vi "DimostratoreCalibrazioni.vi"() -> ()   [LabVIEW 2019]
uses:
  TypeDef/SlugExpiration.ctl
  ByteGSAPIBase/ByteGSAPIBase.lvclass
  TypeDef/CalibrationStates.ctl
  ByteGSAPIBase/FetchCalibration/Converted_Slug_Cluster.ctl
  ByteGSAPIBase/Instruments/Instruments.ctl
  ByteGSAPIBase/CalibrationMeasurements/BodyCalibrazioneMisure.ctl
  aa47c742-c095-4670-bf1f-6b28e4309cef.vi
  <vilib>/numeric/Random Number (Range) I64.vi
  <vilib>/Array/Sort 2D Array - Pop Stack.vi
  <vilib>/Array/Sort 2D Array - Push Stack.vi
  <vilib>/numeric/sub_Random U32.vi
panel:
  in  "Exit":bool
  out "Calibrations":string
  out "Stato":string
  out "Misurazione n.":string
  in  "Cancel":bool
  in  "Approvation":bool
  in  "Avanti":bool
  in  "Repeat":bool
  out "Esito":string
  out "Valore misurato":dbl
  out "Valore di riferimento":dbl
  out "Waveform Chart":i64(graph)
  in  "Start Calibration":bool
  in  "Next":bool
  in  "Previus":bool
  out "Taratura n.":string
  in  "Filtro":enum16{"All", "Expired", "Not Expired"}(ring)
  in  "Slug list":T1[](array[typedef])
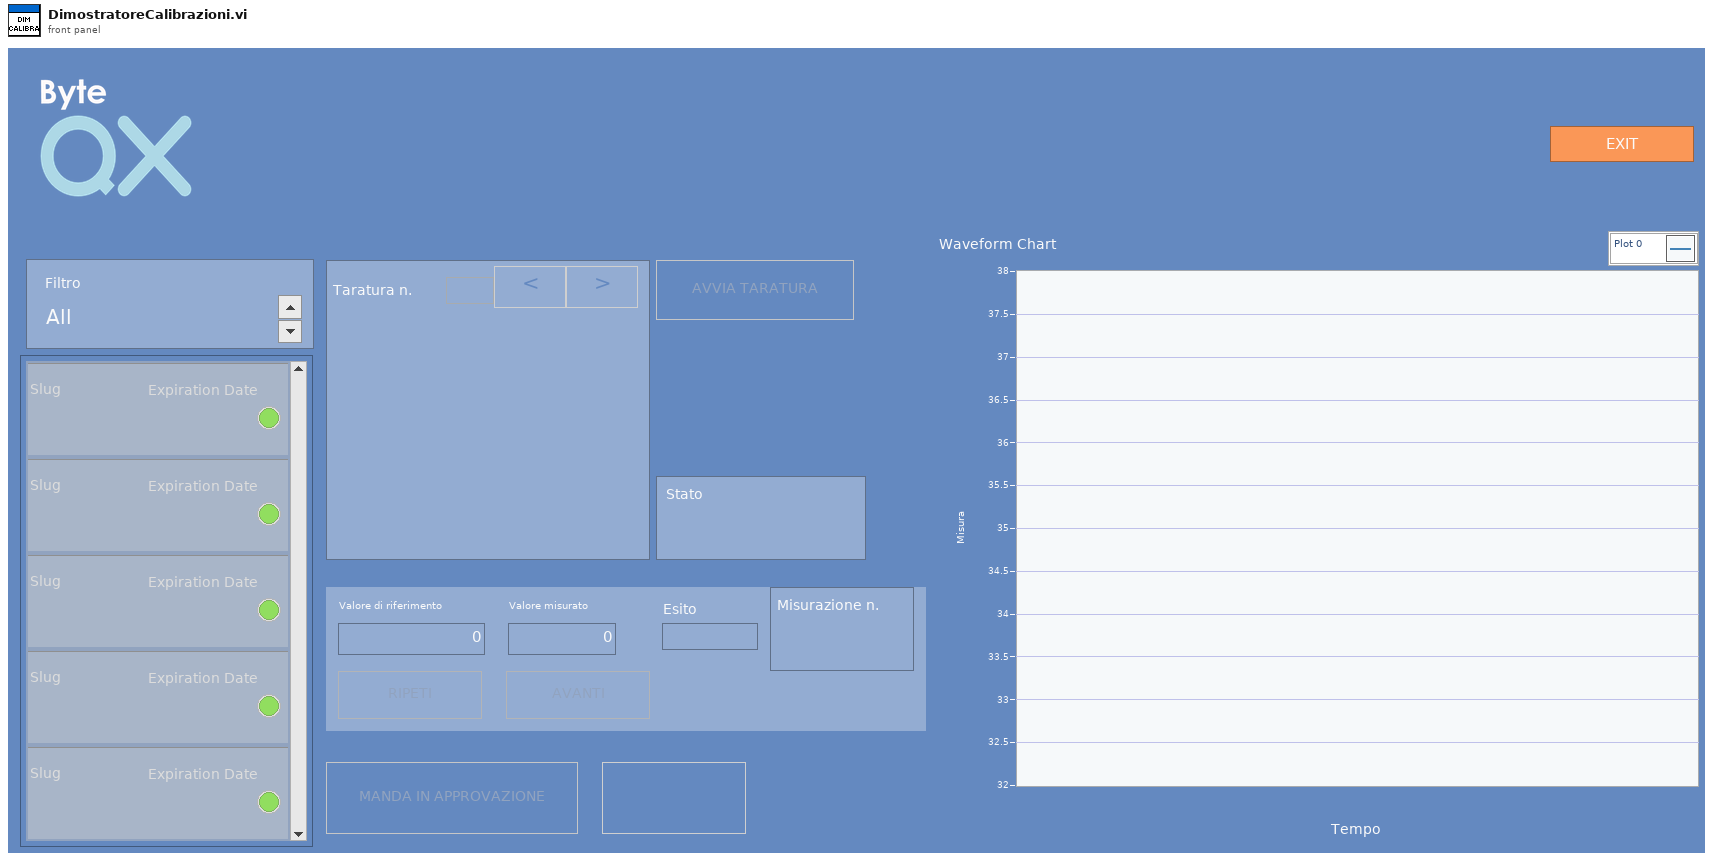
[diagram p1: front panel]
types:
  T1 = typedef "SlugExpiration.ctl" = cluster{"Slug":string, "Expiration Date":string, "Color Box":u32, "Active":bool, "Expired?":bool, "Id":i32}
  T2 = typedef "CalibrationStates.ctl" = enum16{"Init", "Idle", "GetInstruments", "Fetch", "GetCalibrations", "CheckTotalMisurations", "StartCalibration", "ManageCalibration", "AllowApprove", "Approve"}
  T3 = typedef "ByteGSWebAPI.lvlib/ByteGSAPIBase.lvclass/BodyCalibrazioneMisure.ctl" = cluster{"controls":cluster{"id":u16, "descrizione":string, "numero_misure_necessarie":u16, "riferimento_obiettivo":dbl, "mpe_max":dbl, "mpe_min":dbl, "deviazione_standard":dbl, "incertezza":dbl, "numero_misure_effettuate":u32, "temperatura_c":dbl, "umidita":dbl, "strumento_riferimento":cluster{"id":u16, "nome":string}[]}[]}
  T4 = typedef "Instruments.ctl" = cluster{"id":i32, "slug":string, "stabilimento":cluster{"id":dbl}, "categoria":cluster{"id":dbl}, "tipologia_di_visualizzazione":cluster{"id":dbl}, "stato":cluster{"id":dbl}, "descrizione":string, "costruttore":string, "matricola":string, "data_registrazione":string, "intervallo_di_taratura_mesi":dbl, "reparto":string, "campo_misura":string, "risoluzione":dbl, "responsabile_strumento":string, "classe_di_precisione":string, "classificazione":string, "appunti":string, "manuale":string, "foto":string, "riferimento":bool, "qr_hashcode":string, "costo_euro":dbl}
  T5 = typedef "ByteGSWebAPI.lvlib/ByteGSAPIBase.lvclass/Converted_Slug_Cluster.ctl" = cluster{"id":u32, "instrument":string, "name":string, "date":timestamp}
  T6 = cluster{"Esito":refnum<vi>, "Avanti":refnum<vi>, "Repeat":refnum<vi>, "Slug list":refnum<vi>, "Start Calibration":refnum<vi>, "Avanti":refnum<vi>, "Cancel":refnum<vi>, "Approvation":refnum<vi>}
  T7 = cluster{"ByteGSAPIBase in":refnum<class "ByteGSAPIBase.lvclass">, "Instruments_Slug":string[], "All_Instruments_Cals":T5[], "All_Instruments":T4[], "Slug list All":T1[], "Calibrations":T3, "Selected Slug":i32, "Misurazioni":string, "Misurazioni index":i32, "Next State":T2, "Waveform Chart":refnum<vi>, "New Val":dbl, "Id Failed":u32, "Failed?":bool, "Cal Index":i32, "Misurazioni n":string, "Stato":string, "Esito":string, "Misure effettuate":i32, "Calibrations":string}
  T8 = cluster{"id":u16, "descrizione":string, "numero_misure_necessarie":u16, "riferimento_obiettivo":dbl, "mpe_max":dbl, "mpe_min":dbl, "deviazione_standard":dbl, "incertezza":dbl, "numero_misure_effettuate":u32, "temperatura_c":dbl, "umidita":dbl, "strumento_riferimento":cluster{"id":u16, "nome":string}[]}[]
  T9 = cluster{"id":u16, "descrizione":string, "numero_misure_necessarie":u16, "riferimento_obiettivo":dbl, "mpe_max":dbl, "mpe_min":dbl, "deviazione_standard":dbl, "incertezza":dbl, "numero_misure_effettuate":u32, "temperatura_c":dbl, "umidita":dbl, "strumento_riferimento":cluster{"id":u16, "nome":string}[]}
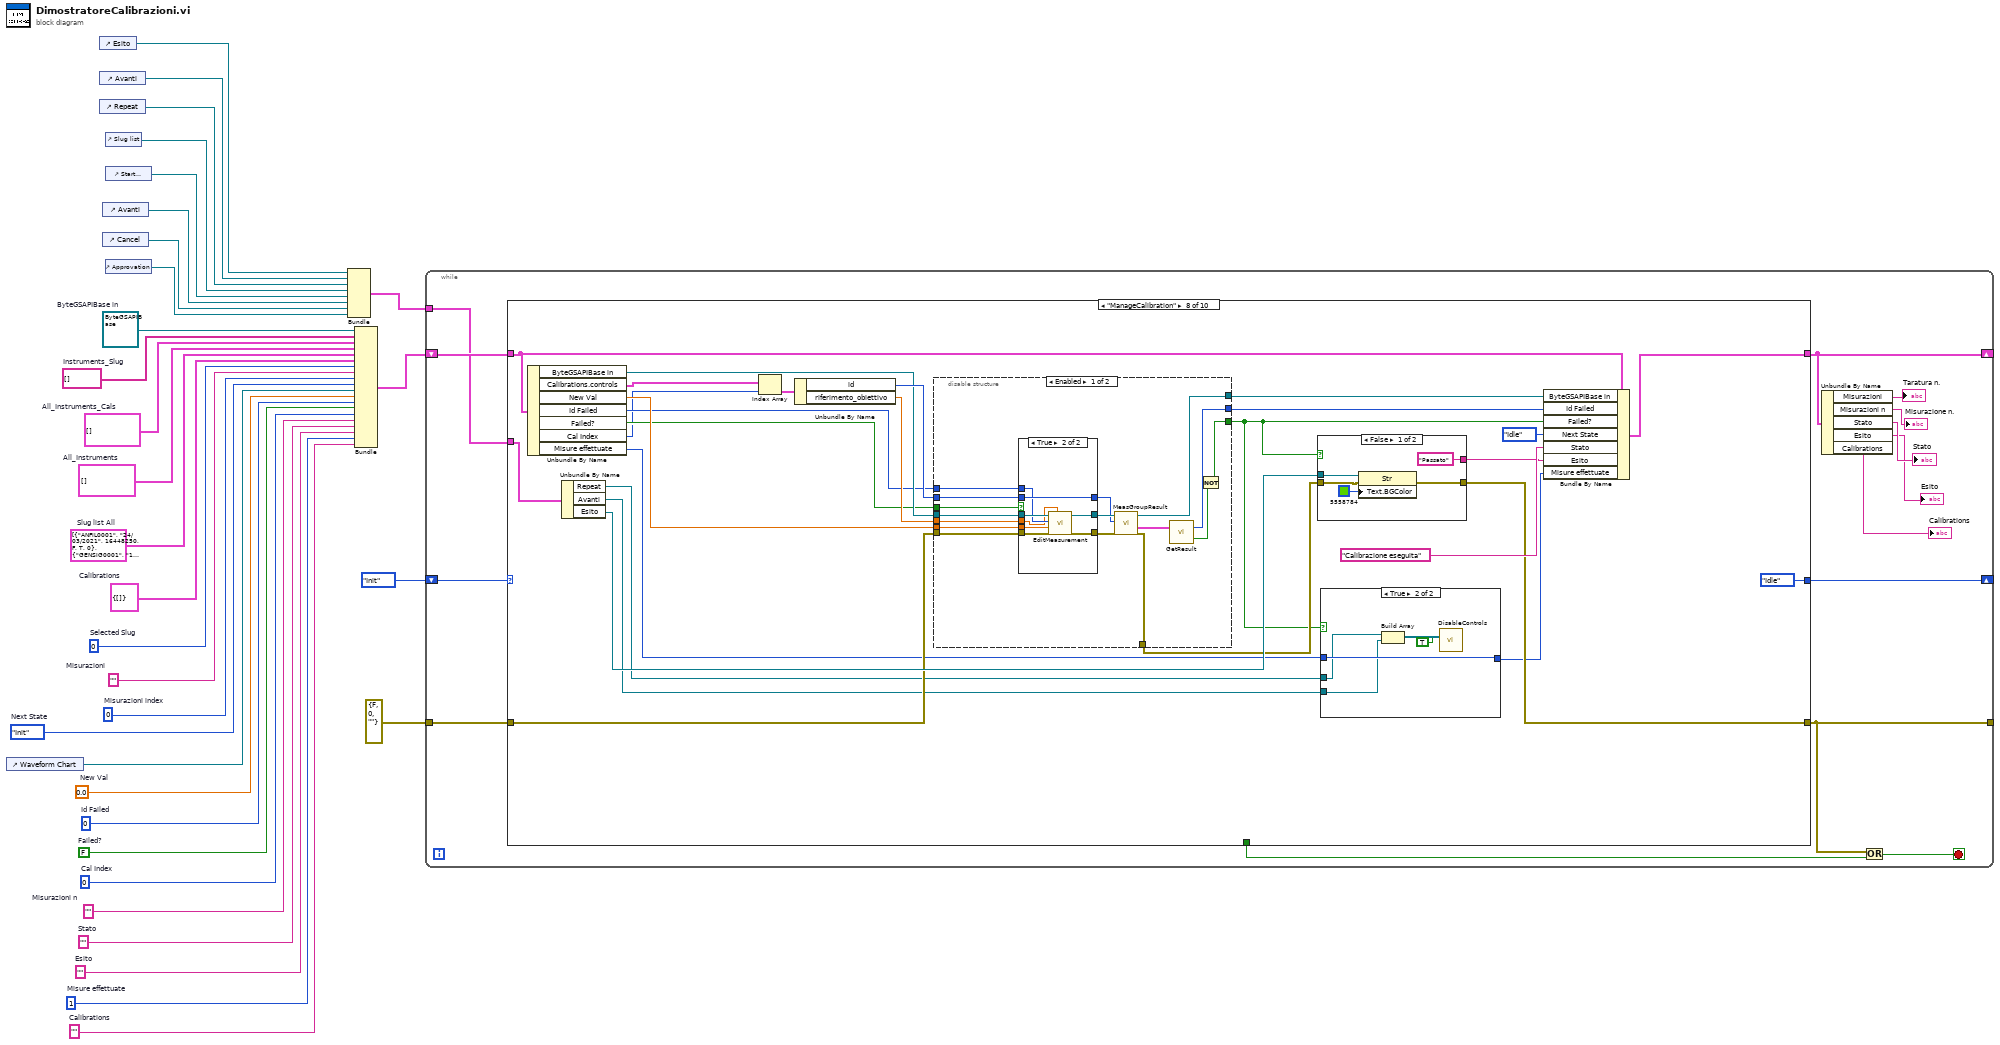
[diagram p0: block diagram]
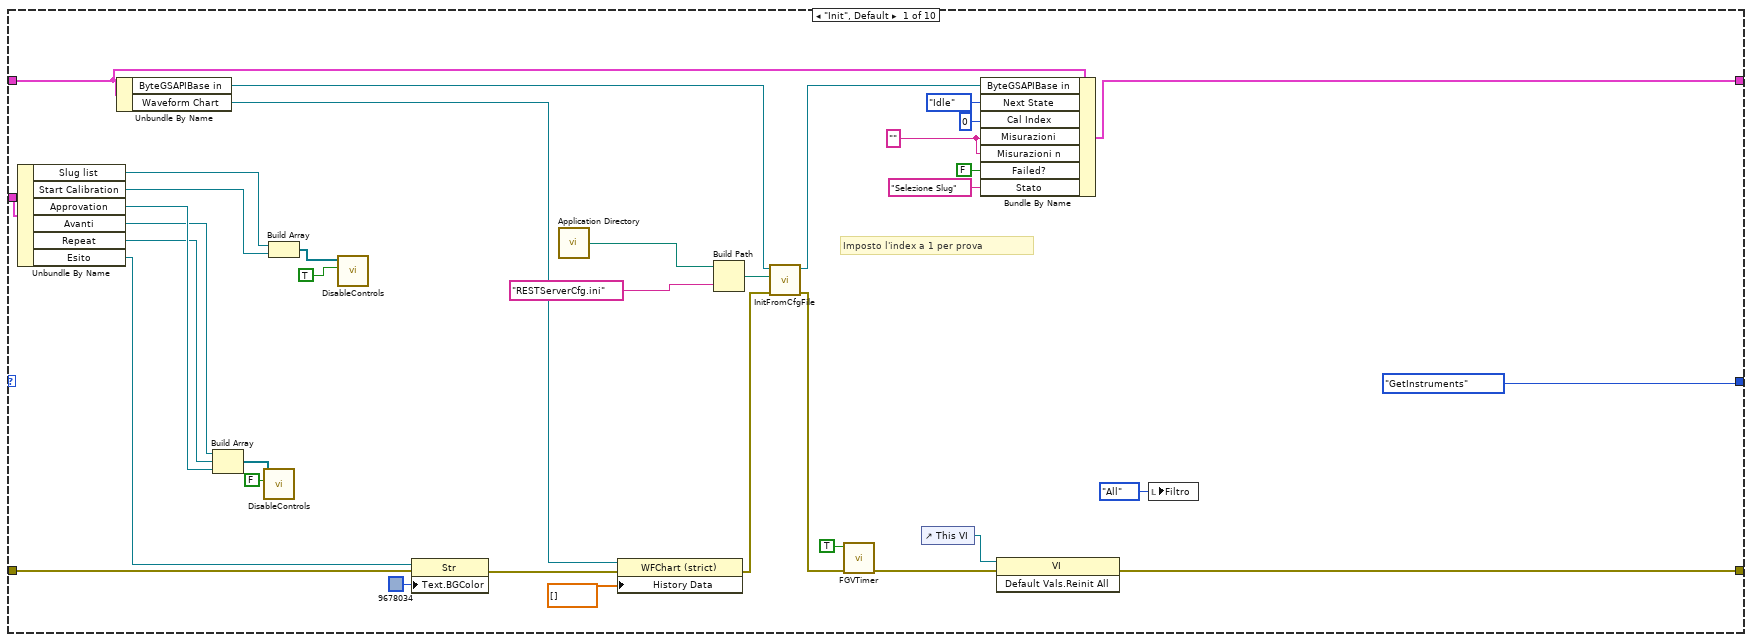
[diagram p2: hidden frame]
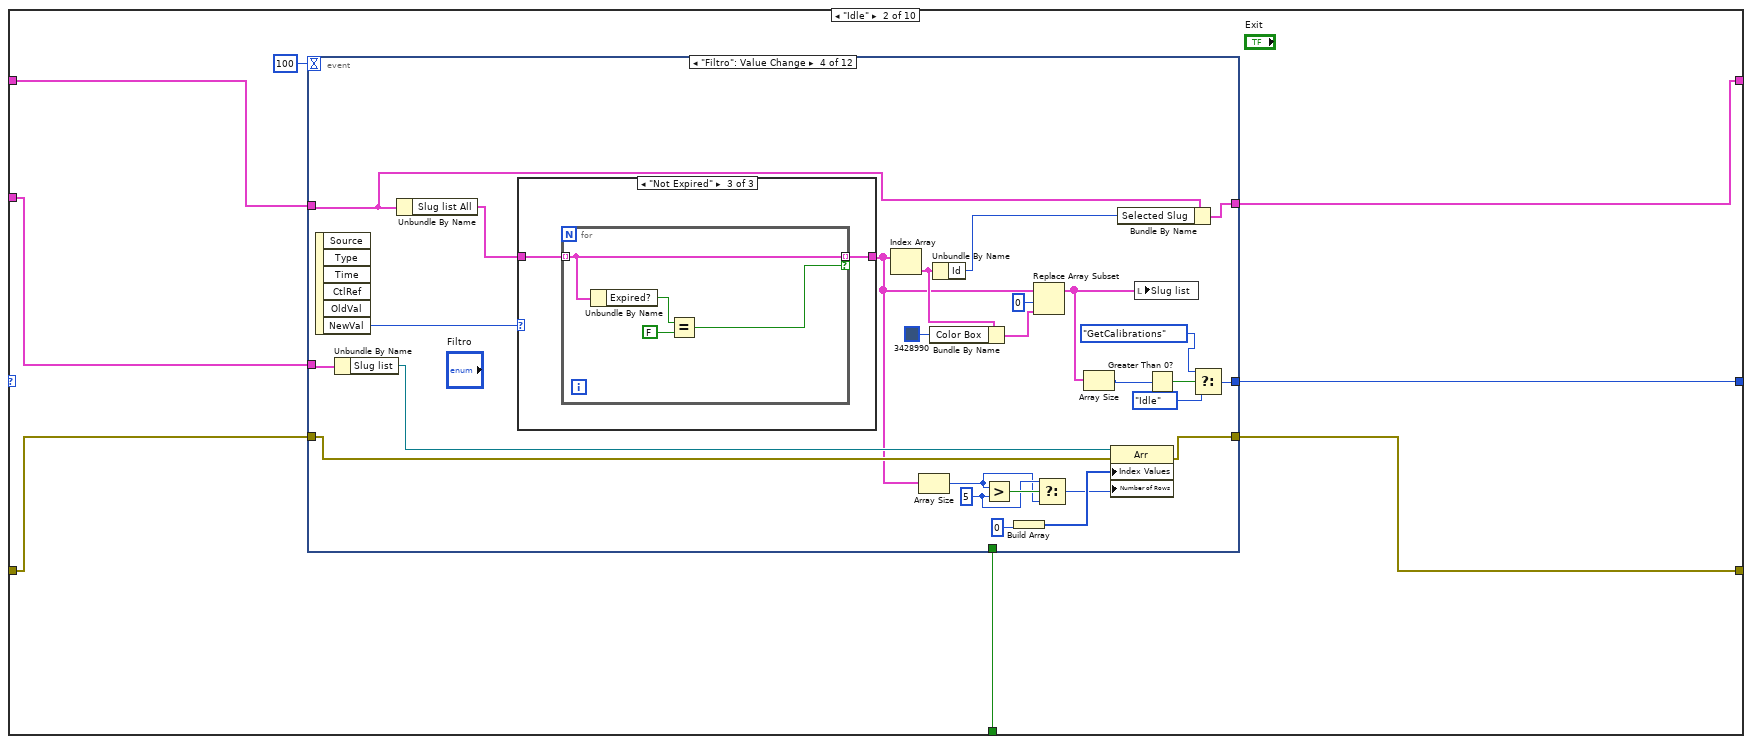
[diagram p3: hidden frame]
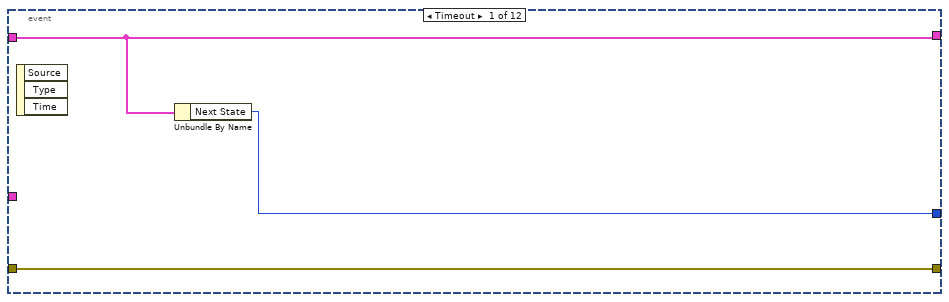
[diagram p4: hidden frame]
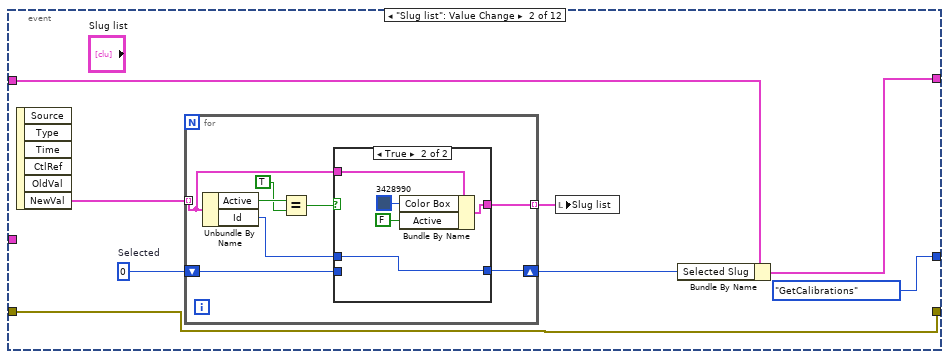
[diagram p5: hidden frame]
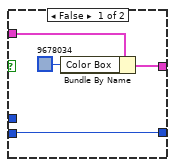
[diagram p6: hidden frame]
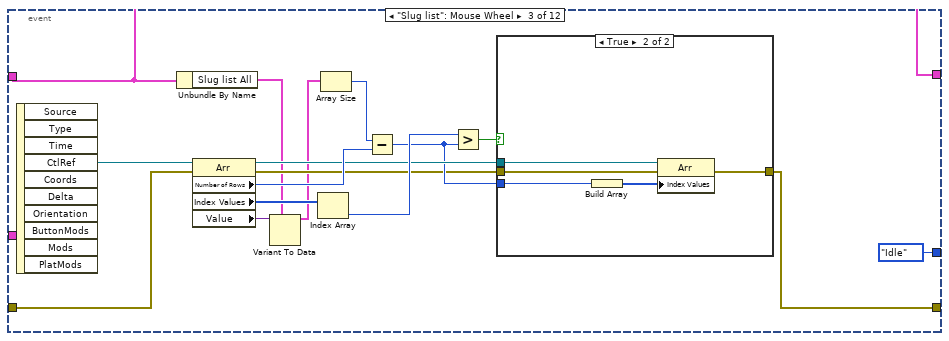
[diagram p7: hidden frame]
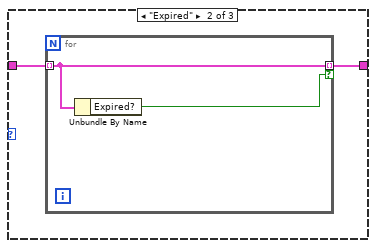
[diagram p10: hidden frame]
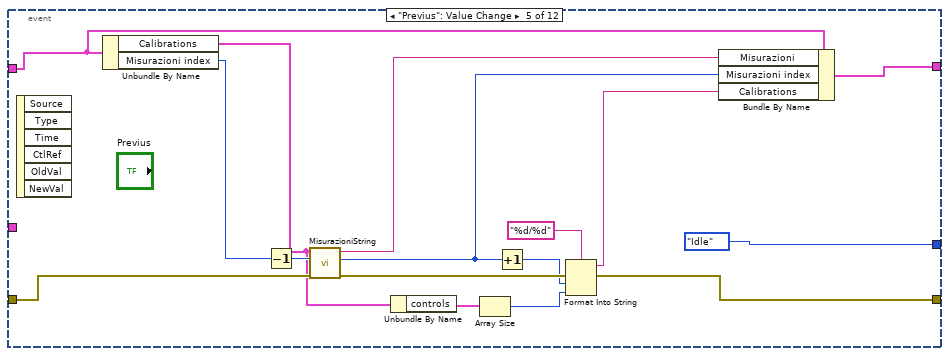
[diagram p11: hidden frame]
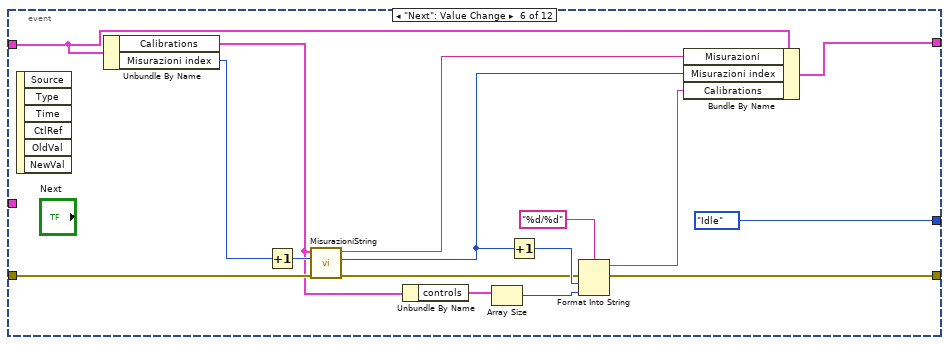
[diagram p12: hidden frame]
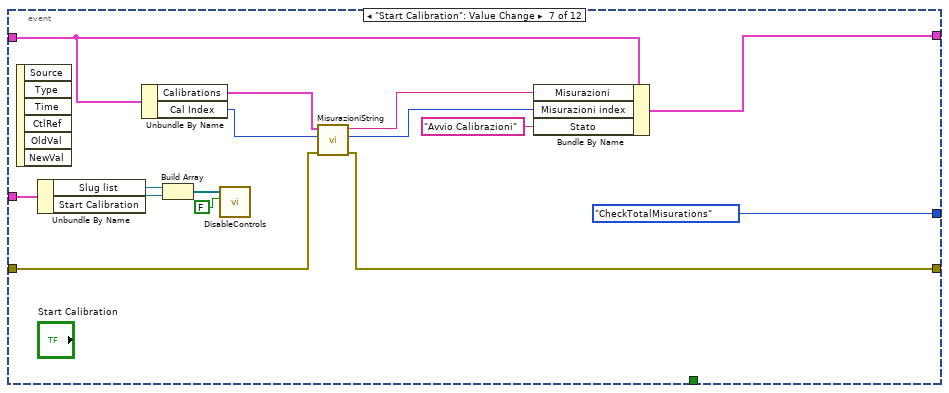
[diagram p13: hidden frame]
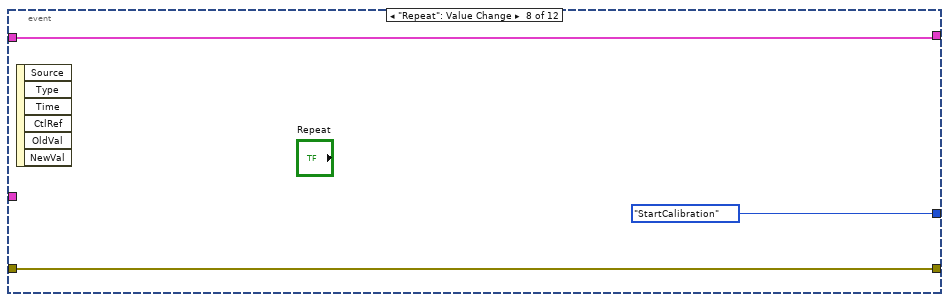
[diagram p14: hidden frame]
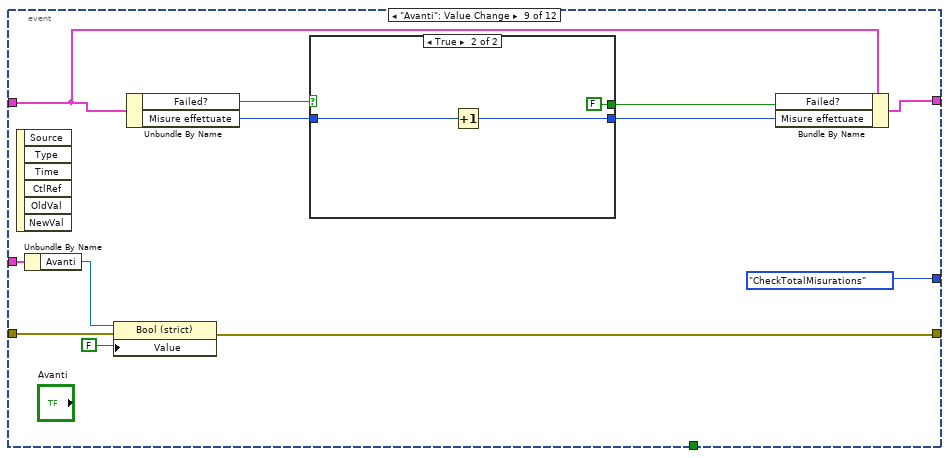
[diagram p15: hidden frame]
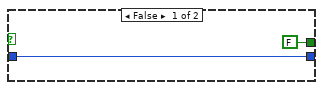
[diagram p16: hidden frame]
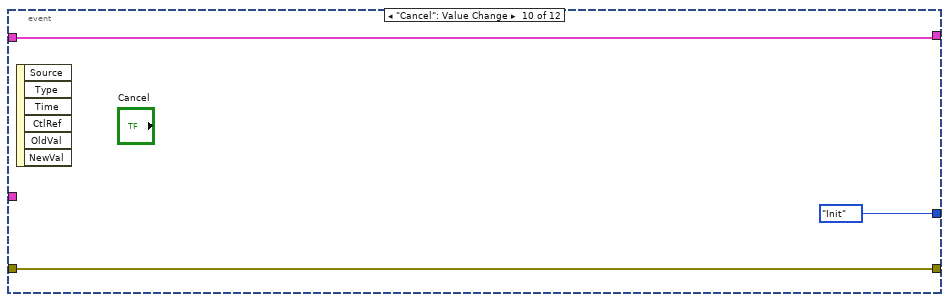
[diagram p17: hidden frame]
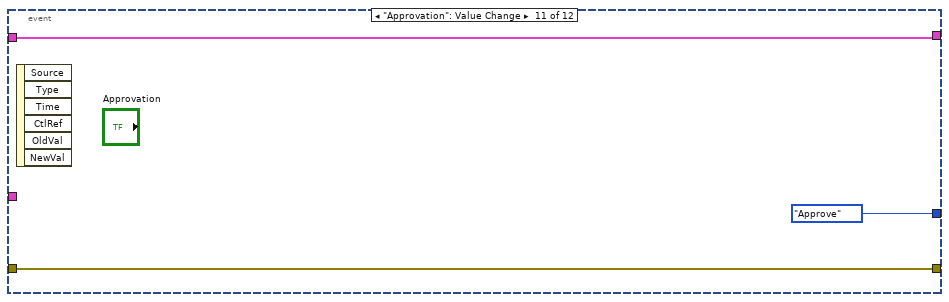
[diagram p18: hidden frame]
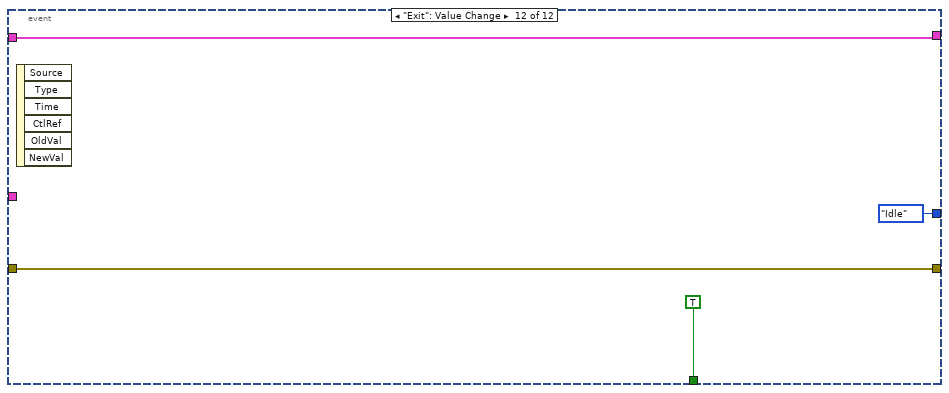
[diagram p19: hidden frame]
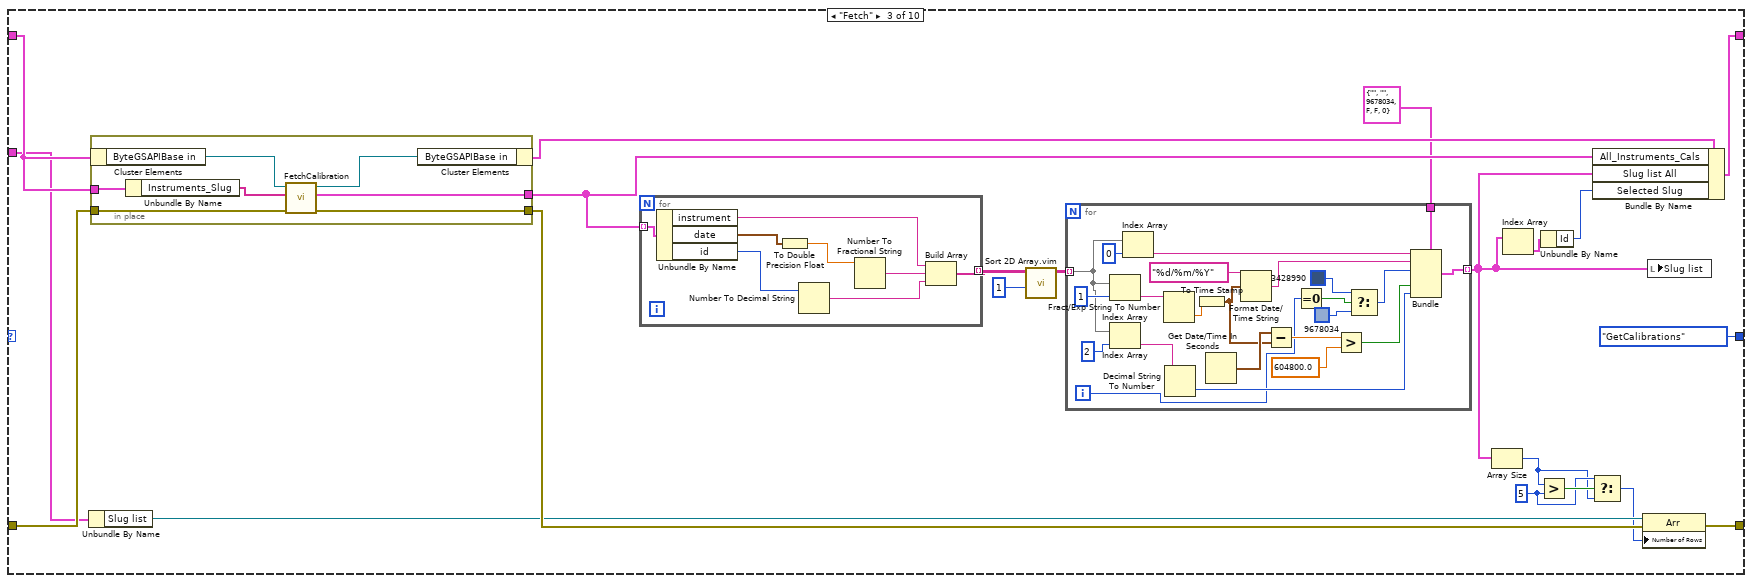
[diagram p20: hidden frame]
diagram:
  w1 = ""  # Calibrations
  w2 = 1  # Misure effettuate
  w4 = ""  # Esito
  w5 = ""  # Stato
  w10 = ""  # Misurazioni n
  w15 = 0  # Cal Index
  w16 = FALSE  # Failed?
  w17 = u32 0  # Id Failed
  w18 = 0.0  # New Val
  w20 = CalibrationStates."Init"  # Next State
  w21 = 0  # Misurazioni index
  w22 = ""  # Misurazioni
  w23 = T1[] [{"Slug"="ANFIL0001", "Expiration Date"="24/03/2021", "Color Box"=16448250, "Active"=FALSE, "Expired?"=TRUE, "Id"=0}, {"Slug"="GENSIG0001", "Expiration Date"="18/05/2021", "Color Box"=16448250, "Active"=FALSE, "Expired?"=TRUE, "Id"=0}, {"Slug"="GENSIG0001", "Expiration Date"="15/09/2021", "Color Box"=16448250, "Active"=FALSE, "Expired?"=TRUE, "Id"=0}, {"Slug"="DIN0001", "Expiration Date"="11/10/2021", "Color Box"=13816530, "Active"=FALSE, "Expired?"=TRUE, "Id"=0}, {"Slug"="DMM0002", "Expiration Date"="20/10/2021", "Color Box"=16448250, "Active"=FALSE, "Expired?"=TRUE, "Id"=0}, {"Slug"="COMP0001", "Expiration Date"="01/12/2021", "Color Box"=16448250, "Active"=FALSE, "Expired?"=TRUE, "Id"=0}, {"Slug"="TORS0002", "Expiration Date"="06/12/2021", "Color Box"=16448250, "Active"=FALSE, "Expired?"=TRUE, "Id"=0}, {"Slug"="CDIND0001", "Expiration Date"="04/03/2022", "Color Box"=16448250, "Active"=FALSE, "Expired?"=TRUE, "Id"=0}, {"Slug"="CALI0004", "Expiration Date"="11/03/2022", "Color Box"=16448250, "Active"=FALSE, "Expired?"=TRUE, "Id"=0}, {"Slug"="CALI0001", "Expiration Date"="10/05/2022", "Color Box"=16448250, "Active"=FALSE, "Expired?"=TRUE, "Id"=0}, {"Slug"="CALI0012", "Expiration Date"="10/05/2022", "Color Box"=16448250, "Active"=FALSE, "Expired?"=TRUE, "Id"=0}, {"Slug"="CALI0011", "Expiration Date"="11/05/2022", "Color Box"=16448250, "Active"=FALSE, "Expired?"=TRUE, "Id"=0}, {"Slug"="CALI0014", "Expiration Date"="04/07/2022", "Color Box"=16448250, "Active"=FALSE, "Expired?"=TRUE, "Id"=0}, {"Slug"="CDIND0001", "Expiration Date"="15/07/2022", "Color Box"=16448250, "Active"=FALSE, "Expired?"=TRUE, "Id"=0}, {"Slug"="CALI0024", "Expiration Date"="11/07/2023", "Color Box"=16448250, "Active"=FALSE, "Expired?"=TRUE, "Id"=0}, {"Slug"="CALI0017", "Expiration Date"="19/09/2023", "Color Box"=16448250, "Active"=FALSE, "Expired?"=TRUE, "Id"=0}, {"Slug"="CALI0020", "Expiration Date"="02/11/2023", "Color Box"=16448250, "Active"=FALSE, "Expired?"=TRUE, "Id"=0}, {"Slug"="CALI0017", "Expiration Date"="03/11/2023", "Color Box"=16448250, "Active"=FALSE, "Expired?"=TRUE, "Id"=0}, {"Slug"="CALI0025", "Expiration Date"="11/11/2023", "Color Box"=16448250, "Active"=FALSE, "Expired?"=TRUE, "Id"=0}, {"Slug"="CLBR0001", "Expiration Date"="30/11/2023", "Color Box"=16448250, "Active"=FALSE, "Expired?"=TRUE, "Id"=0}, {"Slug"="CLBR0001", "Expiration Date"="02/01/2024", "Color Box"=16448250, "Active"=FALSE, "Expired?"=TRUE, "Id"=0}, {"Slug"="CLBR0001", "Expiration Date"="02/01/2024", "Color Box"=16448250, "Active"=FALSE, "Expired?"=TRUE, "Id"=0}, {"Slug"="CLBR0003", "Expiration Date"="04/03/2024", "Color Box"=16448250, "Active"=FALSE, "Expired?"=TRUE, "Id"=0}, {"Slug"="MICP0001", "Expiration Date"="19/03/2024", "Color Box"=16448250, "Active"=FALSE, "Expired?"=TRUE, "Id"=0}, {"Slug"="TERM0002", "Expiration Date"="04/07/2024", "Color Box"=16448250, "Active"=FALSE, "Expired?"=TRUE, "Id"=0}, {"Slug"="ACCEL0008", "Expiration Date"="04/07/2024", "Color Box"=16448250, "Active"=FALSE, "Expired?"=TRUE, "Id"=0}, {"Slug"="ACCEL0008", "Expiration Date"="05/07/2024", "Color Box"=16448250, "Active"=FALSE, "Expired?"=TRUE, "Id"=0}, {"Slug"="ACCEL0008", "Expiration Date"="19/08/2024", "Color Box"=16448250, "Active"=FALSE, "Expired?"=TRUE, "Id"=0}, {"Slug"="TERM0002", "Expiration Date"="15/10/2024", "Color Box"=16448250, "Active"=FALSE, "Expired?"=TRUE, "Id"=0}, {"Slug"="BILA0001", "Expiration Date"="15/10/2024", "Color Box"=16448250, "Active"=FALSE, "Expired?"=TRUE, "Id"=0}, {"Slug"="CLBR0001", "Expiration Date"="15/10/2024", "Color Box"=16448250, "Active"=FALSE, "Expired?"=TRUE, "Id"=0}, {"Slug"="ACCEL0002", "Expiration Date"="15/10/2024", "Color Box"=16448250, "Active"=FALSE, "Expired?"=TRUE, "Id"=0}]  # Slug list All
  w24 = 0  # Selected Slug
  w25 = T3 {"controls"=[]}  # Calibrations
  w26 = T4[] []  # All_Instruments
  w27 = T5[] []  # All_Instruments_Cals
  w28 = string[] []  # Instruments_Slug
  w31 = refnum<class "ByteGSAPIBase.lvclass"> refnum  # ByteGSAPIBase in
  n1 = control-ref of="Waveform Chart"() -> (w19:refnum<vi>)
  n2 = control-ref of="Avanti"() -> (w6:refnum<vi>)
  n3 = control-ref of="Repeat"() -> (w7:refnum<vi>)
  n4 = control-ref of="Esito"() -> (w3:refnum<vi>)
  n5 = control-ref of="Avanti"() -> (w11:refnum<vi>)
  n6 = control-ref of="Cancel"() -> (w12:refnum<vi>)
  n7 = control-ref of="Start Calibration"() -> (w9:refnum<vi>)
  n8 = control-ref of="Approvation"() -> (w13:refnum<vi>)
  n9 = control-ref of="Slug list"() -> (w8:refnum<vi>)
  n10 = Bundle("Esito"=w3, "Avanti"=w6, "Repeat"=w7, "Slug list"=w8, "Start Calibration"=w9, "Avanti"=w11, "Cancel"=w12, "Approvation"=w13) -> (w14:T6)  [unwired: 1 in]
  n11 = Bundle("ByteGSAPIBase in"=w31, "Instruments_Slug"=w28, "All_Instruments_Cals"=w27, "All_Instruments"=w26, "Slug list All"=w23, "Calibrations"=w25, "Selected Slug"=w24, "Misurazioni"=w22, "Misurazioni index"=w21, "Next State"=w20, "Waveform Chart"=w19, "New Val"=w18, "Id Failed"=w17, "Failed?"=w16, "Cal Index"=w15, "Misurazioni n"=w10, "Stato"=w5, "Esito"=w4, "Misure effettuate"=w2, "Calibrations"=w1) -> (w30:T7)  [unwired: 1 in]
  n12 = while {
    shift-right: [w45] -> _
    shift-left: CalibrationStates."Init" -> [w46]
    shift-right: [w42] -> _
    shift-left: w30 -> [w44]
    tunnel: w14 -> [w40]
    tunnel: errorcluster {"status"=FALSE, "code"=0, "source"=""} ("error in (no error)") -> [w43]
    tunnel: [w33] -> _
    stop <- w35 stop-if-true
    n13 = case shown="\"ManageCalibration\"" w46 {
      tunnel: [CalibrationStates."GetInstruments" w88 CalibrationStates."GetCalibrations" CalibrationStates."Fetch" CalibrationStates."Idle" w368 CalibrationStates."Idle" CalibrationStates."Idle" CalibrationStates."Idle" CalibrationStates."Idle"] -> w45
      tunnel: w44 -> [w78 w90 w275 w320 w349 w364 w440 w476 w543 w577]
      tunnel: w43 -> [w48 w87 w274 w322 w350 w366 w425 w462 w546 w576]
      tunnel: [w64 w86 w261 w316 w342 w365 w415 w463 w546 w574] -> w33
      tunnel: [w76 w89 w271 w318 w348 w363 w439 w475 w543 w568] -> w42
      tunnel: w40 -> [w66 w84 w262 _ w335 w367 w429 w468 w552 w573]
      tunnel: [_ w83 _ _ _ _ _ _ _ _] -> w34
      frame "Init", Default {
        w62 = "" ("Misurazioni")
        # "Imposto l'index a 1 per prova"
        n14 = Unbundle By Name(w66) -> ("Slug list"=w60:refnum<vi>, "Start Calibration"=w59:refnum<vi>, "Approvation"=w61:refnum<vi>, "Avanti"=w54:refnum<vi>, "Repeat"=w53:refnum<vi>, "Esito"=w47:refnum<vi>)
        n15 = Unbundle By Name(w78) -> ("ByteGSAPIBase in"=w79:refnum<class "ByteGSAPIBase.lvclass">, "Waveform Chart"=w70:refnum<vi>)
        n16 = Build Array(w54, w53, w61) -> (w56:refnum<vi>[])
        n17 = call "DisableControls.vi"("Visible"=FALSE, "Controls"=w56) -> ()  [unwired: 9 in, 1 out]
        n18 = Build Array(w60, w59) -> (w58:refnum<vi>[])
        n19 = call "DisableControls.vi"("Visible"=TRUE, "Controls"=w58) -> ()  [unwired: 9 in, 1 out]
        n20 = property class="Str"(reference=w47, error in=w48, "Text.BGColor"=u32 9678034 ("Text.Text Colors:BG Color")) -> (error out=w49:errorcluster)  [unwired: 1 out]
        n21 = call <vilib>:"Application Directory.vi"() -> ("Application Directory"=w80:path)
        n22 = property class="WFChart (strict)"(reference=w70, error in=w49, "History Data"=dbl[] []) -> (error out=w69:errorcluster)  [unwired: 1 out]
        n23 = Build Path(base path=w80, name or relative path="RESTServerCfg.ini") -> (appended path=w75:path)
        n24 = call-dynamic "InitFromCfgFile.vi"("error in (no error)"=w69, "configuration file path"=w75, "ByteGSAPIBase in"=w79) -> ("error out"=w73:errorcluster, "ByteGSAPIBase out"=w77:refnum<class "ByteGSAPIBase.lvclass">)  [unwired: 7 in]
        n25 = call "FGVTimer.vi"("error in"=w73, "Reset"=TRUE) -> ("error out"=w65:errorcluster)  [unwired: 7 in, 2 out]
        n26 = control-ref of="This VI"() -> (w63:refnum<vi>)
        n27 = Bundle By Name(cluster=w78, "ByteGSAPIBase in"=w77, "Next State"=CalibrationStates."Idle", "Cal Index"=0, "Misurazioni"=w62, "Misurazioni n"=w62, "Failed?"=FALSE, "Stato"="Selezione Slug") -> (w76:T7)
        n28 = invoke class="VI" method="Default Vals.Reinit All"(reference=w63, error in=w65) -> (error out=w64:errorcluster)  [unwired: 1 in, 2 out]
        n29 = local write "Filtro"(enum16{"All", "Expired", "Not Expired"}."All" ("Filter")) -> ()
      }
      frame "Idle" {
        n30 = event shown="[3] \"Filtro\": Value Change" {
          selector: _ -> [_ _ _ _ _ _ _ _ _ _ _ _]
          dyn-events: _ -> [_ _ _ _ _ _ _ _ _ _ _ _]
          timeout: 100 -> [_ _ _ _ _ _ _ _ _ _ _ _]
          tunnel: w90 -> [w92 w98 w122 w164 w190 w206 w221 w227 w231 w245 w248 w251]
          tunnel: [w92 w96 w122 w163 w189 w204 w218 w227 w230 w245 w248 w251] -> w89
          tunnel: [w91 CalibrationStates."GetCalibrations" CalibrationStates."Idle" w141 CalibrationStates."Idle" CalibrationStates."Idle" CalibrationStates."CheckTotalMisurations" CalibrationStates."StartCalibration" CalibrationStates."CheckTotalMisurations" CalibrationStates."Init" CalibrationStates."Approve" CalibrationStates."Idle"] -> w88
          tunnel: w87 -> [w93 w94 w126 w154 w187 w209 w217 w225 w234 w247 w250 w253]
          tunnel: [w93 w94 w124 w153 w185 w195 w215 w225 w235 w247 w250 w253] -> w86
          tunnel: w84 -> [_ _ _ w156 _ _ w216 _ w236 _ _ _]
          tunnel: [_ _ _ _ _ _ _ _ _ _ _ TRUE] -> w83
          event Timeout {
            n31 = event-data() -> ()  [unwired: 1 in, 3 out]
            n32 = Unbundle By Name(w92) -> ("Next State"=w91:T2)
          }
          event "Slug list": Value Change {
            w99 = 0  # Selected
            n33 = event-data() -> ("NewVal"=w101:T1[])  [unwired: 1 in, 5 out]
            n34 = for {
              tunnel: w101 -> [w106] mode=indexing
              tunnel: [w105] -> w100 mode=indexing
              shift-right: [w103] -> w97
              shift-left: w99 -> [w104]
              n35 = Unbundle By Name(w106) -> ("Active"=w109:bool, "Id"=w102:i32)
              n36 = Equal?(x=w109, y=TRUE) -> (x = y?=w107:bool)
              n37 = case shown="True" w107 {
                tunnel: w106 -> [w112 w118]
                tunnel: [w113 w116] -> w105
                tunnel: w104 -> [w110 _]
                tunnel: [w110 w114] -> w103
                tunnel: w102 -> [_ w114]
                frame False {
                  n38 = Bundle By Name(cluster=w112, "Color Box"=u32 9678034) -> (w113:T1)
                }
                frame True {
                  n39 = Bundle By Name(cluster=w118, "Color Box"=u32 3428990, "Active"=FALSE) -> (w116:T1)
                }
              }
            }
            n40 = local write "Slug list"(w100) -> ()
            n41 = Bundle By Name(cluster=w98, "Selected Slug"=w97) -> (w96:T7)
          }
          event "Slug list": Mouse Wheel {
            n42 = event-data() -> ("CtlRef"=w134:refnum<vi>)  [unwired: 1 in, 9 out]
            n43 = Unbundle By Name(w122) -> ("Slug list All"=w119:T1[])
            n44 = property class="Arr"(reference=w134, error in=w126) -> (reference out=w128:refnum<vi>, error out=w125:errorcluster, "Number of Rows"=w131:u32, "Index Values"=w133:u32[], "Value"=w120:variant)
            n45 = Variant To Data(type=w119, Variant=w120) -> (data=w121:T1[])  [unwired: 1 in, 1 out]
            n46 = Index Array(array=w133) -> (element=w130:u32)  [unwired: 1 in]
            n47 = Array Size(array=w121) -> (size(s)=w132:i32)
            n48 = Subtract(x=w132, y=w131) -> (x-y=w127:u32)
            n49 = Greater?(x=w130, y=w127) -> (0:w129:bool)
            n50 = case shown="True" w129 {
              tunnel: w128 -> [_ w140]
              tunnel: w127 -> [_ w139]
              tunnel: w125 -> [w135 w137]
              tunnel: [w135 w136] -> w124
              frame False {
              }
              frame True {
                n51 = Build Array(w139) -> (w138:u32[])
                n52 = property class="Arr"(reference=w140, error in=w137, "Index Values"=w138) -> (error out=w136:errorcluster)  [unwired: 1 out]
              }
            }
          }
          event "Filtro": Value Change {
            w150 = 5 ("y")
            n53 = event-data() -> ("NewVal"=w166:enum16{"All", "Expired", "Not Expired"})  [unwired: 1 in, 5 out]
            n54 = Unbundle By Name(w156) -> ("Slug list"=w155:refnum<vi>)
            n55 = Unbundle By Name(w164) -> ("Slug list All"=w165:T1[])
            n56 = case shown="\"Not Expired\"" w166 {
              tunnel: w165 -> [w167 w169 w173]
              tunnel: [w167 w168 w172] -> w147
              frame "All" {
              }
              frame "Expired" {
                n57 = for {
                  tunnel: w169 -> [w171] mode=indexing
                  tunnel: [w171] -> w168 mode=indexing if=w170
                  n58 = Unbundle By Name(w171) -> ("Expired?"=w170:bool)
                }
              }
              frame "Not Expired" {
                n59 = for {
                  tunnel: w173 -> [w177] mode=indexing
                  tunnel: [w177] -> w172 mode=indexing if=w174
                  n60 = Unbundle By Name(w177) -> ("Expired?"=w176:bool)
                  n61 = Equal?(x=w176, y=FALSE) -> (x = y?=w174:bool)
                }
              }
            }
            n62 = Index Array(array=w147) -> (element=w161:T1)  [unwired: 1 in]
            n63 = Array Size(array=w147) -> (size(s)=w149:i32)
            n64 = Bundle By Name(cluster=w161, "Color Box"=u32 3428990) -> (w159:T1)
            n65 = Unbundle By Name(w161) -> ("Id"=w162:i32)
            n66 = Greater?(x=w149, y=w150) -> (0:w151:bool)
            n67 = Build Array(0) -> (w157:i32[])
            n68 = Replace Array Subset(array=w147, new element=w159, index=0) -> (w144:T1[])
            n69 = Select(t=w150, s=w151, f=w149) -> (s? t:f=w148:i32)
            n70 = Array Size(array=w144) -> (size(s)=w145:i32)
            n71 = property class="Arr"(reference=w155, error in=w154, "Index Values"=w157, "Number of Rows"=w148) -> (error out=w153:errorcluster)  [unwired: 1 out]
            n72 = Bundle By Name(cluster=w164, "Selected Slug"=w162) -> (w163:T7)
            n73 = local write "Slug list"(w144) -> ()
            n74 = Greater Than 0?(x=w145) -> (x > 0?=w146:bool)
            n75 = Select(t=CalibrationStates."GetCalibrations", s=w146, f=CalibrationStates."Idle") -> (s? t:f=w141:T2)
          }
          event "Previus": Value Change {
            n76 = event-data() -> ()  [unwired: 1 in, 6 out]
            n77 = Unbundle By Name(w190) -> ("Calibrations"=w181:T3, "Misurazioni index"=w192:i32)
            n78 = Decrement(x=w192) -> (x-1=w193:i32)
            n79 = call "MisurazioniString.vi"("error in (no error)"=w187, "index"=w193, "Calibration data"=w181) -> ("error out"=w186:errorcluster, "index"=w183:i32, "String"=w191:string)  [unwired: 6 in]
            n80 = Unbundle By Name(w181) -> ("controls"=w180:T8)
            n81 = Array Size(array=w180) -> (size(s)=w179:i32)
            n82 = Increment(x=w183) -> (x+1=w182:i32)
            n83 = Format Into String(format string="%d/%d", error in=w186, w182, w179) -> (resulting string=w178:string, error out=w185:errorcluster)  [unwired: 1 in]
            n84 = Bundle By Name(cluster=w190, "Misurazioni"=w191, "Misurazioni index"=w183, "Calibrations"=w178) -> (w189:T7)
          }
          event "Next": Value Change {
            n85 = event-data() -> ()  [unwired: 1 in, 6 out]
            n86 = Unbundle By Name(w206) -> ("Calibrations"=w200:T3, "Misurazioni index"=w207:i32)
            n87 = Increment(x=w207) -> (x+1=w208:i32)
            n88 = call "MisurazioniString.vi"("error in (no error)"=w209, "index"=w208, "Calibration data"=w200) -> ("error out"=w198:errorcluster, "index"=w197:i32, "String"=w205:string)  [unwired: 6 in]
            n89 = Unbundle By Name(w200) -> ("controls"=w196:T8)
            n90 = Array Size(array=w196) -> (size(s)=w199:i32)
            n91 = Increment(x=w197) -> (x+1=w201:i32)
            n92 = Format Into String(format string="%d/%d", error in=w198, w201, w199) -> (resulting string=w194:string, error out=w195:errorcluster)  [unwired: 1 in]
            n93 = Bundle By Name(cluster=w206, "Misurazioni"=w205, "Misurazioni index"=w197, "Calibrations"=w194) -> (w204:T7)
          }
          event "Start Calibration": Value Change {
            n94 = event-data() -> ()  [unwired: 1 in, 6 out]
            n95 = Unbundle By Name(w216) -> ("Slug list"=w214:refnum<vi>, "Start Calibration"=w213:refnum<vi>)
            n96 = Unbundle By Name(w221) -> ("Calibrations"=w223:T3, "Cal Index"=w222:i32)
            n97 = Build Array(w214, w213) -> (w212:refnum<vi>[])
            n98 = call "DisableControls.vi"("Visible"=FALSE, "Controls"=w212) -> ()  [unwired: 9 in, 1 out]
            n99 = call "MisurazioniString.vi"("error in (no error)"=w217, "index"=w222, "Calibration data"=w223) -> ("error out"=w215:errorcluster, "index"=w219:i32, "String"=w220:string)  [unwired: 6 in]
            n100 = Bundle By Name(cluster=w221, "Misurazioni"=w220, "Misurazioni index"=w219, "Stato"="Avvio Calibrazioni") -> (w218:T7)
          }
          event "Repeat": Value Change {
            n101 = event-data() -> ()  [unwired: 1 in, 6 out]
          }
          event "Avanti": Value Change {
            n102 = event-data() -> ()  [unwired: 1 in, 6 out]
            n103 = Unbundle By Name(w236) -> ("Avanti"=w238:refnum<vi>)
            n104 = property class="Bool (strict)"(reference=w238, error in=w234, "Value"=FALSE) -> (error out=w235:errorcluster)  [unwired: 1 out]
            n105 = Unbundle By Name(w231) -> ("Failed?"=w233:bool, "Misure effettuate"=w232:i32)
            n106 = case shown="True" w233 {
              tunnel: w232 -> [w241 w244]
              tunnel: [w241 w243] -> w229
              tunnel: [FALSE FALSE] -> w228
              frame False {
              }
              frame True {
                n107 = Increment(x=w244) -> (x+1=w243:i32)
              }
            }
            n108 = Bundle By Name(cluster=w231, "Failed?"=w228, "Misure effettuate"=w229) -> (w230:T7)
          }
          event "Cancel": Value Change {
            n109 = event-data() -> ()  [unwired: 1 in, 6 out]
          }
          event "Approvation": Value Change {
            n110 = event-data() -> ()  [unwired: 1 in, 6 out]
          }
          event "Exit": Value Change {
            n111 = event-data() -> ()  [unwired: 1 in, 6 out]
          }
        }
      }
      frame "Fetch" {
        w257 = 5 ("y")
        n112 = Unbundle By Name(w262) -> ("Slug list"=w259:refnum<vi>)
        n113 = in-place {
          in-place-border: w274 -> [w312]
          in-place-border: [w311] -> w260
          in-place-border: [w310] -> w267
          in-place-border: w275 -> [w308]
          n114 = in-place-cluster #1(w275) -> ("ByteGSAPIBase in"=w309:refnum<class "ByteGSAPIBase.lvclass">)
          n115 = Unbundle By Name(w308) -> ("Instruments_Slug"=w307:string[])
          n116 = call "FetchCalibration.vi"("error in (no error)"=w312, "Instruments"=w307, "ByteGSAPIBase in"=w309) -> ("error out"=w311:errorcluster, "Instruments"=w310:T5[], "ByteGSAPIBase out"=w313:refnum<class "ByteGSAPIBase.lvclass">)  [unwired: 6 in]
          n117 = in-place-cluster #1("ByteGSAPIBase in"=w313) -> (w272:T7)
        }
        n118 = for {
          tunnel: w267 -> [w306] mode=indexing
          tunnel: [w305] -> w270 mode=indexing
          n119 = Unbundle By Name(w306) -> ("instrument"=w304:string, "date"=w303:timestamp, "id"=w300:u32)
          n120 = To Double Precision Float(number=w303) -> (double precision float=w302:dbl)
          n121 = Number To Decimal String(number=w300) -> (decimal integer string=w299:string)  [unwired: 1 in]
          n122 = Number To Fractional String(number=w302) -> (F-format string=w301:string)  [unwired: 3 in]
          n123 = Build Array(w304, w301, w299) -> (w305:string[])
        }
        n124 = call "Sort 2D Array.vim"("index"=1, "2D array"=w270) -> ("sorted 2D array"=w268:string[][])  [unwired: 8 in, 1 out]
        n125 = for {
          tunnel: w268 -> [w283] mode=indexing
          tunnel: T1 {"Slug"="", "Expiration Date"="", "Color Box"=9678034, "Active"=FALSE, "Expired?"=FALSE, "Id"=0} ("Slug list 2") -> [w298]
          tunnel: [w290] -> w263 mode=indexing
          i -> [w280]
          n126 = Index Array(array=w283, index=1) -> (element=w294:string)
          n127 = Index Array(array=w283, index=2) -> (element=w282:string)
          n128 = Index Array(array=w283, index=0) -> (element=w296:string)
          n129 = Fract/Exp String To Number(string=w294) -> (number=w293:dbl)  [unwired: 3 in, 1 out]
          n130 = Decimal String To Number(string=w282) -> (number=w281:i32)  [unwired: 2 in, 1 out]
          n131 = To Time Stamp(1:w293) -> (0:w285:timestamp)
          n132 = Get Date/Time In Seconds() -> (seconds since 1Jan1904=w286:timestamp)
          n133 = Format Date/Time String(time format string (%c)="%d/%m/%Y", seconds (now)=w285) -> (date/time string=w291:string)  [unwired: 1 in]
          n134 = Subtract(x=w286, y=w285) -> (x-y=w289:dbl)
          n135 = Equal To 0?(x=w280) -> (x = 0?=w279:bool)
          n136 = Greater?(x=w289, y=604800.0) -> (0:w287:bool)
          n137 = Select(t=u32 3428990 ("Color Box"), s=w279, f=u32 9678034 ("Color Box")) -> (s? t:f=w276:u32)
          n138 = Bundle(cluster=w298, "Slug"=w296, "Expiration Date"=w291, "Color Box"=w276, "Expired?"=w287, "Id"=w281) -> (w290:T1)  [unwired: 1 in]
        }
        n139 = Array Size(array=w263) -> (size(s)=w256:i32)
        n140 = Index Array(array=w263) -> (element=w265:T1)  [unwired: 1 in]
        n141 = Greater?(x=w256, y=w257) -> (0:w258:bool)
        n142 = Unbundle By Name(w265) -> ("Id"=w264:i32)
        n143 = Select(t=w257, s=w258, f=w256) -> (s? t:f=w255:i32)
        n144 = Bundle By Name(cluster=w272, "All_Instruments_Cals"=w267, "Slug list All"=w263, "Selected Slug"=w264) -> (w271:T7)
        n145 = property class="Arr"(reference=w259, error in=w260, "Number of Rows"=w255) -> (error out=w261:errorcluster)  [unwired: 1 out]
        n146 = local write "Slug list"(w263) -> ()
      }
      frame "GetInstruments" {
        n147 = Unbundle By Name(w320) -> ("ByteGSAPIBase in"=w321:refnum<class "ByteGSAPIBase.lvclass">)
        n148 = call "InstrumentsList.vi"("error in (no error)"=w322, "ByteGSAPIBase in"=w321) -> ("error out"=w316:errorcluster, "Array"=w315:T4[], "ByteGSAPIBase out"=w319:refnum<class "ByteGSAPIBase.lvclass">)  [unwired: 7 in]
        n149 = for {
          tunnel: w315 -> [w324] mode=indexing
          tunnel: [w323] -> w314 mode=indexing
          n150 = Unbundle By Name(w324) -> ("slug"=w323:string)
        }
        n151 = Bundle By Name(cluster=w320, "ByteGSAPIBase in"=w319, "All_Instruments"=w315, "Instruments_Slug"=w314) -> (w318:T7)
      }
      frame "GetCalibrations" {
        n152 = Unbundle By Name(w335) -> ("Start Calibration"=w332:refnum<vi>)
        n153 = Unbundle By Name(w349) -> ("ByteGSAPIBase in"=w351:refnum<class "ByteGSAPIBase.lvclass">, "Selected Slug"=w352:i32)
        n154 = call "ExecutingCalibration.vi"("error in (no error)"=w350, "calibration_id"=w352, "ByteGSAPIBase in"=w351) -> ("error out"=w346:errorcluster, "Calibration data"=w343:T3, "ByteGSAPIBase out"=w347:refnum<class "ByteGSAPIBase.lvclass">)  [unwired: 6 in]
        n155 = call "MisurazioniString.vi"("error in (no error)"=w346, "index"=0, "Calibration data"=w343) -> ("error out"=w326:errorcluster, "index"=w329:i32, "String"=w345:string)  [unwired: 6 in]
        n156 = Unbundle By Name(w343) -> ("controls"=w336:T8)
        n157 = for {
          tunnel: w336 -> [w360] mode=indexing
          tunnel: [w354] -> w333
          stop <- w354 stop-if-true
          n158 = Unbundle By Name(w360) -> ("numero_misure_necessarie"=w359:u16, "numero_misure_effettuate"=w358:u32)
          n159 = Less Or Equal?(x=w359, y=w358) -> (x <= y?=w357:bool)
          n160 = Select(t=FALSE, s=w357, f=TRUE) -> (s? t:f=w354:bool)
        }
        n161 = Build Array(w332) -> (w334:refnum<vi>[])
        n162 = call "DisableControls.vi"("Visible"=w333, "Controls"=w334) -> ()  [unwired: 9 in, 1 out]
        n163 = Index Array(array=w336) -> (element=w339:T9)  [unwired: 1 in]
        n164 = Array Size(array=w336) -> (size(s)=w330:i32)
        n165 = Increment(x=w329) -> (x+1=w328:i32)
        n166 = Unbundle By Name(w339) -> ("numero_misure_effettuate"=w337:u32, "numero_misure_necessarie"=w338:u16)
        n167 = Format Into String(format string="%d/%d", error in=w326, w328, w330) -> (resulting string=w327:string, error out=w325:errorcluster)  [unwired: 1 in]
        n168 = Format Into String(format string="%d/%d", error in=w325, w337, w338) -> (resulting string=w340:string, error out=w342:errorcluster)  [unwired: 1 in]
        n169 = Bundle By Name(cluster=w349, "ByteGSAPIBase in"=w347, "Calibrations"=w343, "Misurazioni"=w345, "Misurazioni index"=w329, "Misurazioni n"=w340, "Misure effettuate"=w337, "Calibrations"=w327) -> (w348:T7)
      }
      frame "CheckTotalMisurations" {
        n170 = Unbundle By Name(w367) -> ()  [unwired: 1 out]
        n171 = Unbundle By Name(w364) -> ("Calibrations"=w373:T3, "Cal Index"=w362:i32, "Misure effettuate"=w361:i32)
        n172 = Unbundle By Name(w373) -> ("controls"=w372:T8)
        n173 = Index Array(array=w372, index=w362) -> (element=w371:T9)
        n174 = Unbundle By Name(w371) -> ("numero_misure_necessarie"=w370:u16)
        n175 = Less Or Equal?(x=w370, y=w361) -> (x <= y?=w369:bool)
        n176 = case shown="True" w369 {
          tunnel: [CalibrationStates."StartCalibration" w385] -> w368
          tunnel: w366 -> [w375 w394]
          tunnel: [w375 w380] -> w365
          tunnel: w364 -> [w374 w396]
          tunnel: [w374 w391] -> w363
          tunnel: w362 -> [_ _]
          frame False {
          }
          frame True {
            n177 = Unbundle By Name(w396) -> ("Misure effettuate"=w398:i32, "Cal Index"=w389:i32, "Waveform Chart"=w393:refnum<vi>, "Calibrations"=w402:T3)
            n178 = Unbundle By Name(w402) -> ("controls"=w390:T8)
            n179 = Index Array(array=w390, index=w389) -> (element=w401:T9)
            n180 = Unbundle By Name(w401) -> ("numero_misure_necessarie"=w400:u16)
            n181 = property class="WFChart (strict)"(reference=w393, error in=w394, "History Data"=dbl[] []) -> (error out=w392:errorcluster)  [unwired: 1 out]
            n182 = Less Or Equal?(x=w400, y=w398) -> (x <= y?=w399:bool)
            n183 = case shown="True" w399 {
              tunnel: w389 -> [w408 w413]
              tunnel: [w408 w412] -> w406
              tunnel: w398 -> [w407 _]
              tunnel: [w407 w409] -> w397
              tunnel: w390 -> [_ w411]
              frame False {
              }
              frame True {
                n184 = Increment(x=w413) -> (x+1=w412:i32)
                n185 = Index Array(array=w411, index=w412) -> (element=w410:T9)
                n186 = Unbundle By Name(w410) -> ("numero_misure_effettuate"=w409:u32)
              }
            }
            n187 = Array Size(array=w390) -> (size(s)=w377:i32)
            n188 = Decrement(x=w377) -> (x-1=w384:i32)
            n189 = call "MisurazioniString.vi"("error in (no error)"=w392, "index"=w406, "Calibration data"=w402) -> ("error out"=w381:errorcluster, "index"=w378:i32, "String"=w405:string)  [unwired: 6 in]
            n190 = Less Or Equal?(x=w384, y=w389) -> (x <= y?=w388:bool)
            n191 = Increment(x=w378) -> (x+1=w382:i32)
            n192 = Format Into String(format string="%d/%d", error in=w381, w382, w377) -> (resulting string=w379:string, error out=w380:errorcluster)  [unwired: 1 in]
            n193 = Bundle By Name(cluster=w396, "Misure effettuate"=w397, "Cal Index"=w406, "Misurazioni"=w405, "Misurazioni index"=w378, "Id Failed"=u32 0, "Failed?"=FALSE, "Calibrations"=w379) -> (w391:T7)
            n194 = Select(t=CalibrationStates."AllowApprove", s=w388, f=CalibrationStates."CheckTotalMisurations") -> (s? t:f=w385:T2)
          }
        }
      }
      frame "StartCalibration" {
        n195 = Unbundle By Name(w429) -> ("Esito"=w428:refnum<vi>, "Avanti"=w417:refnum<vi>, "Repeat"=w414:refnum<vi>)
        n196 = Build Array(w417, w414) -> (w419:refnum<vi>[])
        n197 = property class="Str"(reference=w428, error in=w425, "Text.BGColor"=u32 9678034 ("Text.Text Colors:BG Color")) -> (error out=w426:errorcluster)  [unwired: 1 out]
        n198 = Unbundle By Name(w440) -> ("Calibrations"=w444:T3, "New Val"=w437:dbl, "Cal Index"=w424:i32, "Misure effettuate"=w421:i32)  [unwired: 1 out]
        n199 = call "DisableControls.vi"("Visible"=FALSE, "Controls"=w419) -> ()  [unwired: 9 in, 1 out]
        n200 = Unbundle By Name(w444) -> ("controls"=w416:T8)
        n201 = call "FGVTimer.vi"("error in"=w426) -> ("error out"=w433:errorcluster, "Elapsed?"=w441:bool)  [unwired: 8 in, 1 out]
        n202 = Index Array(array=w416, index=w424) -> (element=w443:T9)
        n203 = Unbundle By Name(w443) -> ("riferimento_obiettivo"=w435:dbl)
        "Valore di riferimento" <- w435
        n204 = Index Array(array=w416, index=w424) -> (element=w423:T9)
        n205 = Unbundle By Name(w423) -> ("numero_misure_necessarie"=w422:u16)
        n206 = case shown="False" w441 {
          tunnel: w435 -> [w451 _]
          tunnel: [CalibrationStates."StartCalibration" CalibrationStates."ManageCalibration"] -> w438
          tunnel: [w445 w454] -> w436
          tunnel: w437 -> [_ w454]
          frame False {
            n207 = Quotient & Remainder(x=w451, y=10.0) -> (floor(x/y)=w450:dbl)  [unwired: 1 out]
            n208 = Add(x=w451, y=w450) -> (x+y=w449:dbl)
            n209 = Subtract(x=w451, y=w450) -> (x-y=w446:dbl)
            n210 = To Quad Integer(1:w449) -> (0:w448:i64)
            n211 = To Quad Integer(1:w446) -> (0:w447:i64)
            n212 = call-poly <vilib>:"Random Number (Range).vi"("lower bound (-100)"=w447, "upper bound (100)"=w448) -> ("number"=w445:i64)  [unwired: 9 in]
            "Waveform Chart" <- w445
          }
          frame True {
          }
        }
        "Valore misurato" <- w436
        n213 = Increment(x=w421) -> (x+1=w420:i32)
        n214 = Format Into String(format string="%d/%d", error in=w433, w420, w422) -> (resulting string=w432:string, error out=w415:errorcluster)  [unwired: 1 in]
        n215 = Bundle By Name(cluster=w440, "Next State"=w438, "New Val"=w436, "Misurazioni n"=w432, "Stato"="Calibrazione in corso", "Esito"="...") -> (w439:T7)
      }
      frame "ManageCalibration" {
        n216 = Unbundle By Name(w476) -> ("ByteGSAPIBase in"=w479:refnum<class "ByteGSAPIBase.lvclass">, "Calibrations.controls"=w482:T8, "New Val"=w478:dbl, "Id Failed"=w474:u32, "Failed?"=w471:bool, "Cal Index"=w461:i32, "Misure effettuate"=w459:i32)
        n217 = Unbundle By Name(w468) -> ("Repeat"=w457:refnum<vi>, "Avanti"=w458:refnum<vi>, "Esito"=w465:refnum<vi>)
        n218 = Index Array(array=w482, index=w461) -> (element=w481:T9)
        n219 = Unbundle By Name(w481) -> ("id"=w480:u16, "riferimento_obiettivo"=w477:dbl)
        n220 = disable-structure shown="Enabled" {
          disable-tunnel: w480 -> [w521 _]
          disable-tunnel: w479 -> [w520 w539]
          disable-tunnel: w478 -> [w519 w541]
          disable-tunnel: w477 -> [w518 w542]
          disable-tunnel: w462 -> [w517 w540]
          disable-tunnel: [w513 w540] -> w464
          disable-tunnel: w474 -> [w511 _]
          disable-tunnel: [w510 w539] -> w473
          disable-tunnel: [w509 _] -> w472
          disable-tunnel: w471 -> [w508 _]
          disable-tunnel: [w506 w537] -> w460
          frame Enabled {
            n221 = case shown="True" w508 {
              tunnel: w520 -> [w528 w536]
              tunnel: w518 -> [w527 w529]
              tunnel: w519 -> [w526 w534]
              tunnel: w517 -> [w525 w535]
              tunnel: [w524 w532] -> w516
              tunnel: w521 -> [w522 w531]
              tunnel: [w523 w533] -> w515
              tunnel: [w522 w531] -> w514
              tunnel: w511 -> [_ w530]
              frame False {
                n222 = call-dynamic "AddMeasurement.vi"("measurement_group id"=w522, "error in (no error)"=w525, "misura_strumento"=w526, "misura_riferimento"=w527, "ByteGSAPIBase in"=w528) -> ("error out"=w524:errorcluster, "ByteGSAPIBase out"=w523:refnum<class "ByteGSAPIBase.lvclass">)  [unwired: 4 in, 1 out]
              }
              frame True {
                n223 = call-dynamic "EditMeasurement.vi"("objective measure"=w529, "error in (no error)"=w535, "instrument measure"=w534, "measurement id"=w530, "ByteGSAPIBase in"=w536) -> ("error out"=w532:errorcluster, "ByteGSAPIBase out"=w533:refnum<class "ByteGSAPIBase.lvclass">)  [unwired: 4 in, 1 out]
              }
            }
            n224 = call "MeasGroupResult.vi"("error in (no error)"=w516, "measurement_group_id"=w514, "ByteGSAPIBase in"=w515) -> ("error out"=w513:errorcluster, "measurements"=w512:cluster{"id":u32, "passed":bool}[], "ByteGSAPIBase out"=w510:refnum<class "ByteGSAPIBase.lvclass">)  [unwired: 5 in, 1 out]
            n225 = call "GetResult.vi"("measurements"=w512) -> ("passed"=w507:bool, "id"=w509:u32)  [unwired: 1 in]
            n226 = Not(x=w507) -> (.not. x?=w506:bool)
          }
          frame Disabled {
            n227 = Equal?(x=w542, y=w541) -> (x = y?=w538:bool)
            n228 = Not(x=w538) -> (.not. x?=w537:bool)
          }
        }
        n229 = case shown="False" w460 {
          tunnel: ["Passato" ("Esito") "Fallito" ("Esito")] -> w466
          tunnel: w465 -> [w499 w503]
          tunnel: w464 -> [w497 w502]
          tunnel: [w496 w501] -> w463
          frame False {
            n230 = property class="Str"(reference=w499, error in=w497, "Text.BGColor"=u32 5558784 ("Text.Text Colors:BG Color")) -> (error out=w496:errorcluster)  [unwired: 1 out]
          }
          frame True {
            n231 = property class="Str"(reference=w503, error in=w502, "Text.BGColor"=u32 16737380 ("Text.Text Colors:BG Color")) -> (error out=w501:errorcluster)  [unwired: 1 out]
          }
        }
        n232 = case shown="True" w460 {
          tunnel: w459 -> [w490 w495]
          tunnel: [w489 w495] -> w456
          tunnel: w457 -> [w484 w492]
          tunnel: w458 -> [w483 w491]
          frame False {
            n233 = Build Array(w483) -> (w486:refnum<vi>[])
            n234 = Build Array(w484) -> (w488:refnum<vi>[])
            n235 = Increment(x=w490) -> (x+1=w489:i32)
            n236 = call "DisableControls.vi"("Visible"=FALSE, "Controls"=w488) -> ()  [unwired: 9 in, 1 out]
            n237 = call "DisableControls.vi"("Visible"=TRUE, "Controls"=w486) -> ()  [unwired: 9 in, 1 out]
          }
          frame True {
            n238 = Build Array(w492, w491) -> (w494:refnum<vi>[])
            n239 = call "DisableControls.vi"("Visible"=TRUE, "Controls"=w494) -> ()  [unwired: 9 in, 1 out]
          }
        }
        n240 = Bundle By Name(cluster=w476, "ByteGSAPIBase in"=w473, "Id Failed"=w472, "Failed?"=w460, "Next State"=CalibrationStates."Idle", "Stato"="Calibrazione eseguita", "Esito"=w466, "Misure effettuate"=w456) -> (w475:T7)
      }
      frame "AllowApprove" {
        n241 = Unbundle By Name(w552) -> ("Repeat"=w551:refnum<vi>, "Approvation"=w549:refnum<vi>, "Avanti"=w550:refnum<vi>)
        n242 = Unbundle By Name(w543) -> ("Calibrations.controls"=w544:T8, "Misure effettuate"=w548:i32, "Cal Index"=w547:i32)
        n243 = Array Size(array=w544) -> (size(s)=w559:i32)
        n244 = Decrement(x=w559) -> (x-1=w558:i32)
        n245 = Index Array(array=w544, index=w547) -> (element=w557:T9)
        n246 = Less Or Equal?(x=w558, y=w547) -> (x <= y?=w554:bool)
        n247 = Unbundle By Name(w557) -> ("numero_misure_necessarie"=w556:u16)
        n248 = Equal?(x=w548, y=w556) -> (x = y?=w555:bool)
        n249 = And(x=w555, y=w554) -> (x .and. y?=w553:bool)
        n250 = case shown="True" w553 {
          tunnel: w549 -> [_ w563]
          tunnel: w550 -> [_ w566]
          tunnel: w551 -> [_ w560]
          frame False {
          }
          frame True {
            n251 = Build Array(w563) -> (w562:refnum<vi>[])
            n252 = Build Array(w566, w560) -> (w565:refnum<vi>[])
            n253 = call "DisableControls.vi"("Visible"=TRUE, "Controls"=w562) -> ()  [unwired: 9 in, 1 out]
            n254 = call "DisableControls.vi"("Visible"=FALSE, "Controls"=w565) -> ()  [unwired: 9 in, 1 out]
          }
        }
      }
      frame "Approve" {
        n255 = Unbundle By Name(w573) -> ("Approvation"=w572:refnum<vi>)
        n256 = Build Array(w572) -> (w571:refnum<vi>[])
        n257 = call "DisableControls.vi"("Visible"=FALSE, "Controls"=w571) -> ()  [unwired: 9 in, 1 out]
        n258 = disable-structure shown="Enabled" {
          disable-tunnel: w577 -> [w578 w589]
          disable-tunnel: w576 -> [w581 w588]
          disable-tunnel: [w580 w589] -> w569
          disable-tunnel: [w579 w588] -> w574
          frame Enabled {
            n259 = in-place {
              in-place-border: w578 -> [w585]
              in-place-border: [w584] -> w579
              in-place-border: w581 -> [w582]
              n260 = in-place-cluster #2(w578) -> ("ByteGSAPIBase in"=w587:refnum<class "ByteGSAPIBase.lvclass">)
              n261 = Unbundle By Name(w585) -> ("Selected Slug"=w583:i32)
              n262 = call "RequestApproval.vi"("error in (no error)"=w582, "calibration_id"=w583, "ByteGSAPIBase in"=w587) -> ("error out"=w584:errorcluster, "ByteGSAPIBase out"=w586:refnum<class "ByteGSAPIBase.lvclass">)  [unwired: 6 in, 1 out]
              n263 = in-place-cluster #2("ByteGSAPIBase in"=w586) -> (w580:T7)
            }
          }
          frame Disabled {
          }
        }
        n264 = Bundle By Name(cluster=w569, "Stato"="Approvazione inviata") -> (w568:T7)
      }
    }
    n265 = Unbundle By Name(w42) -> ("Misurazioni"=→"Taratura n.":string, "Misurazioni n"=→"Misurazione n.":string, "Stato"=→"Stato":string, "Esito"=→"Esito":string, "Calibrations"=→"Calibrations":string)
    n266 = Or(x=w33, y=w34) -> (x .or. y?=w35:bool)
  }
